vi "IHM_checkVariables_loop.vi"() -> ()   [LabVIEW 2009]
panel:
  in  "attente (ms)":u32
  out "index":i32
  in  "stop":bool
  out "InputCh0":dbl
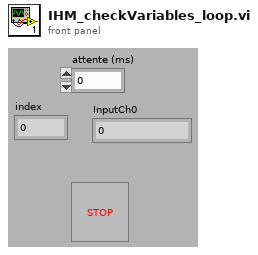
[diagram p1: front panel]
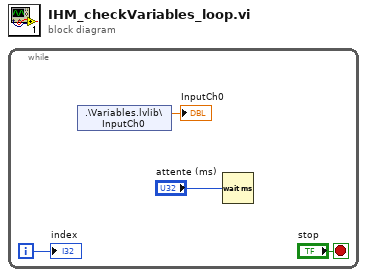
[diagram p0: block diagram]
diagram:
  n1 = while {
    i -> [w2]
    stop <- "stop" stop-if-true
    n2 = shared-variable ".\\Variables.lvlib\\InputCh0"() -> (→"InputCh0":dbl)  [unwired: 1 in, 1 out]
    n3 = Wait (ms)(milliseconds to wait="attente (ms)") -> ()  [unwired: 1 out]
    "index" <- w2
  }
